vi "Lockin.vi"(7 "Initialize?":bool, 8 "error in (no error)":errorcluster, 10 "data":waveform(dbl)[](array[waveform]), 11 "Lock-in settings":T1={"Sine Frequency, Hz"=0.0, "Time constant, s"=0.12500000000000006, "Low-pass filter"=enum."No filtering", "Output representation"=enum."Real/Imaginary", "Phases, deg"=[], "Low-pass filter Order"=1, "Decimating factor"=1, "Samples to Read"=10000, "Post-filter decimation"=1, "Blocks to average"=1, "Trig delay, points"=0, "Harmonics per channel"=[], "Amplitude scale"=enum."RMS"} {"Time constant, s" format="%.1e"}) -> (0 "error out":errorcluster, 2 "signal(s) out":waveform(dbl)[](array[waveform]), 3 "Lock-in settings out":T1={"Sine Frequency, Hz"=0.0, "Time constant, s"=0.12500000000000006, "Low-pass filter"=enum."No filtering", "Output representation"=enum."Real/Imaginary", "Phases, deg"=[], "Low-pass filter Order"=1, "Decimating factor"=1, "Samples to Read"=10000, "Post-filter decimation"=1, "Blocks to average"=1, "Trig delay, points"=0, "Harmonics per channel"=[], "Amplitude scale"=enum."RMS"} {"Time constant, s" format="%.1e"})   [LabVIEW 2015]
uses:
  Controls/Lockin Settings.ctl
  Controls/Harmonics per channel.ctl
  <vilib>/Analysis/NI_AALPro.lvlib
  <vilib>/Analysis/2dsp.llb/Decimate (single shot, DBL).vi
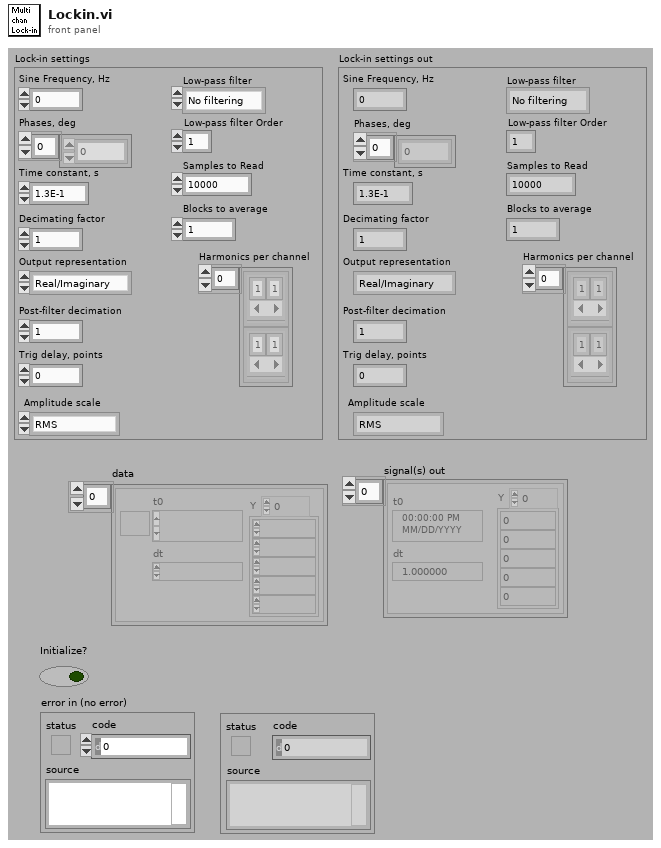
[diagram p1: front panel]
types:
  T1 = typedef "Lockin Settings.ctl" = cluster{"Sine Frequency, Hz":dbl, "Time constant, s":dbl, "Low-pass filter":enum16{"No filtering", "Butterworth", "Bessel"}, "Output representation":enum16{"Real/Imaginary", "Polar"}, "Phases, deg":dbl[], "Low-pass filter Order":i32, "Decimating factor":i32, "Samples to Read":i32, "Post-filter decimation":i32, "Blocks to average":i32, "Trig delay, points":i32, "Harmonics per channel":T2, "Amplitude scale":enum16{"Amplitude", "RMS", "Peak-to-Peak"}}
  T2 = typedef "Harmonics per channel.ctl" = cluster{"Harmonics":i32[]}[]
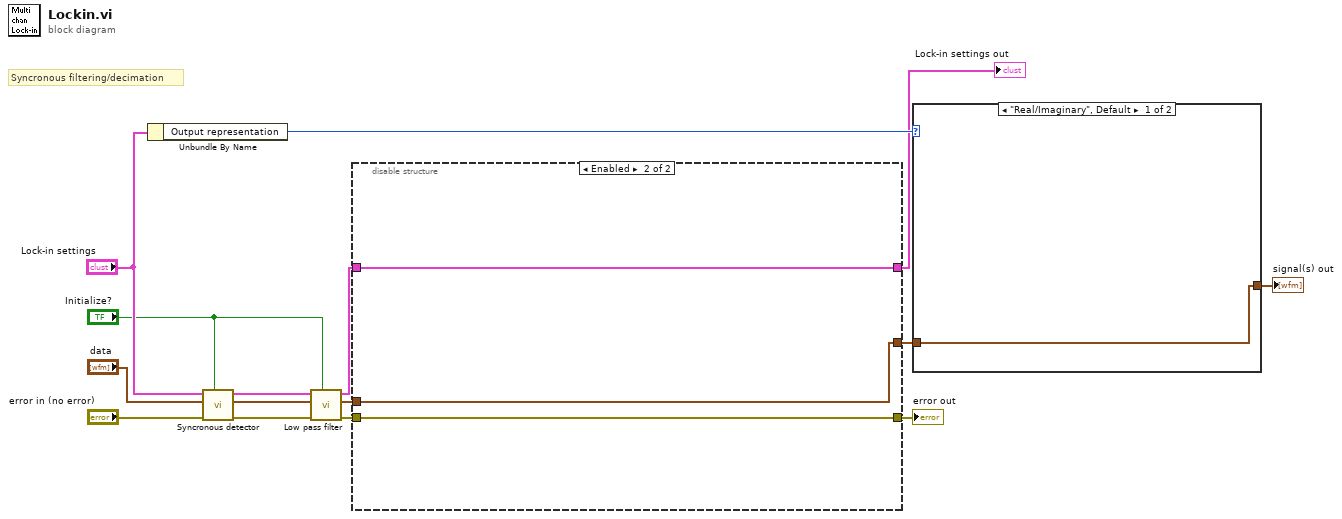
[diagram p0: block diagram]
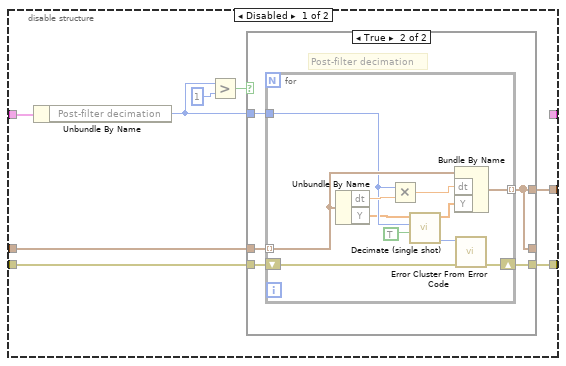
[diagram p2: hidden frame]
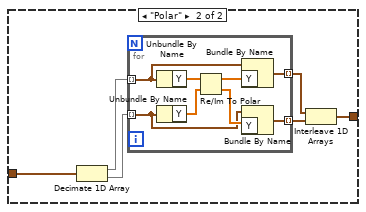
[diagram p4: hidden frame]
diagram:
  # "Syncronous filtering/decimation"
  n1 = Unbundle By Name("Lock-in settings") -> ("Output representation"=w14:enum16{"Real/Imaginary", "Polar"})
  n2 = call "Syncronous detector.vi"("Initialize?"="Initialize?", "error in (no error)"="error in (no error)", "data"="data", "Lock-in settings"="Lock-in settings") -> ("error out"=w6:errorcluster, "signal(s) out"=w8:waveform(dbl)[], "Lock-in settings out"=w7:T1)  [unwired: 5 in]
  n3 = call "Low pass filter.vi"("error in (no error)"=w6, "data"=w8, "Lock-in settings"=w7, "Initialize?"="Initialize?") -> ("error out"=w10:errorcluster, "signal(s) out"=w11:waveform(dbl)[], "Lock-in settings out"=w2:T1)  [unwired: 5 in]
  n4 = disable-structure shown="Enabled" {
    disable-tunnel: [w21 w42] -> w13
    disable-tunnel: [w20 w44] -> w12
    disable-tunnel: w11 -> [w19 w42]
    disable-tunnel: w10 -> [w18 w44]
    disable-tunnel: w2 -> [w17 w43]
    disable-tunnel: [_ w43] -> w3
    frame Disabled {
      n5 = Unbundle By Name(w17) -> ("Post-filter decimation"=w22:i32)
      n6 = Greater?(x=w22, y=1) -> (0:w16:bool)
      n7 = case shown="True" w16 {
        tunnel: w22 -> [_ w30]
        tunnel: w19 -> [w25 w29]
        tunnel: [w25 w28] -> _
        tunnel: [w25 w28] -> w21
        tunnel: w18 -> [w24 w27]
        tunnel: [w24 w26] -> w20
        frame False {
        }
        frame True {
          # "Post-filter decimation"
          n8 = for {
            tunnel: w30 -> [w38]
            tunnel: w29 -> [w40] mode=indexing
            tunnel: [w34] -> w28 mode=indexing
            shift-right: [w31] -> w26
            shift-left: w27 -> [w32]
            n9 = Unbundle By Name(w40) -> ("dt"=w39:dbl, "Y"=w35:dbl[])
            n10 = Multiply(x=w38, y=w39) -> (x*y=w37:dbl)
            n11 = call-poly <vilib>:"Decimate (single shot).vi"("averaging"=TRUE, "decimating factor"=w38, "X"=w35) -> ("error"=w33:i32, "Decimated Array"=w36:dbl[])  [unwired: 7 out]
            n12 = Bundle By Name(cluster=w40, "dt"=w37, "Y"=w36) -> (w34:waveform(dbl))
            n13 = call <vilib>:"Error Cluster From Error Code.vi"("error in (no error)"=w32, "error code (0)"=w33) -> ("error out"=w31:errorcluster)  [unwired: 1 in, 6 out]
          }
        }
      }
    }
    frame Enabled {
    }
  }
  "error out" <- w12
  "Lock-in settings out" <- w3
  n14 = case shown="\"Real/Imaginary\", Default" w14 {
    tunnel: w13 -> [w45 w49]
    tunnel: [w45 w46] -> w15
    frame "Real/Imaginary", Default {
    }
    frame "Polar" {
      n15 = Decimate 1D Array(w49) -> (w51:waveform(dbl)[], w50:waveform(dbl)[])
      n16 = for {
        tunnel: w51 -> [w56] mode=indexing
        tunnel: w50 -> [w52] mode=indexing
        tunnel: [w55] -> w48 mode=indexing
        tunnel: [w53] -> w47 mode=indexing
        n17 = Unbundle By Name(w56) -> ("Y"=w59:dbl[])
        n18 = Unbundle By Name(w52) -> ("Y"=w58:dbl[])
        n19 = Re/Im To Polar(2:w58, 3:w59) -> (0:w54:dbl[], 1:w57:dbl[])
        n20 = Bundle By Name(cluster=w56, "Y"=w57) -> (w55:waveform(dbl))
        n21 = Bundle By Name(cluster=w52, "Y"=w54) -> (w53:waveform(dbl))
      }
      n22 = Interleave 1D Arrays(w48, w47) -> (w46:waveform(dbl)[])
    }
  }
  "signal(s) out" <- w15
